vi "Get Timeout.vi"(8 "error in (no error)":errorcluster, 11 "SwipeScrollListbox in":refnum<class "SwipeScrollListbox.lvclass">) -> (0 "error out":errorcluster, 2 "Timeout":i32, 3 "SwipeScrollListbox out":refnum<class "SwipeScrollListbox.lvclass">)   [LabVIEW 2019, in "SwipeScrollListbox.lvclass"]
uses:
  SwipeScrollListbox.lvclass
  SwipeScrollListbox.lvclass/SwipeScrollListbox.ctl
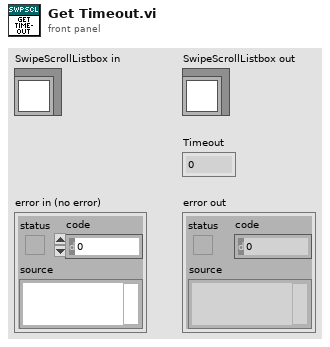
[diagram p1: front panel]
types:
  T1 = typedef "SwipeScrollListbox.lvclass/State Data.ctl" = cluster{"Timeout":i32, "Time":timestamp, "Y":i32, "Slow Distance":i32, "Rate":dbl, "Row Selected":i32}
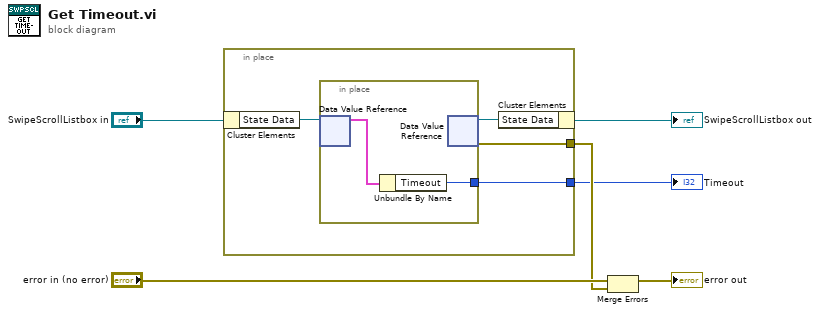
[diagram p0: block diagram]
diagram:
  n1 = in-place {
    in-place-border: [w8] -> w1
    in-place-border: [w7] -> w3
    n2 = in-place-cluster #1("SwipeScrollListbox in") -> ("State Data"=w10:refnum<data-value>)
    n3 = in-place {
      in-place-border: [w11] -> w8
      n4 = in-place-dvr #2(w10) -> (w12:T1)  [unwired: 1 out]
      n5 = Unbundle By Name(w12) -> ("Timeout"=w11:i32)
      n6 = in-place-dvr #2() -> (w9:refnum<data-value>, w7:errorcluster)  [unwired: 1 in]
    }
    n7 = in-place-cluster #1("State Data"=w9) -> (→"SwipeScrollListbox out":refnum<class "SwipeScrollListbox.lvclass">)
  }
  "Timeout" <- w1
  n8 = Merge Errors("error in (no error)", w3) -> (→"error out":errorcluster)
